vi "Day_File_Plotter.vi"() -> ()   [LabVIEW 2010]
uses:
  Anemometry/Anemometry Sub Vis/Globals/Constants_global.vi
panel:
  in  "Reload":bool
  out "Setup exists?":bool
  out "Plot 3 status":string
  out "Plot 2 status":string
  out "Plot 1 status":string
  out "Change Scale?":bool
  out "Min Memory":timestamp
  out "Max Memory":timestamp
  in  "Show Full Time?":bool
  in  "Max Time":timestamp format="%<%H:%M\n%x>T"
  in  "Min Time":timestamp format="%<%H:%M\n%x>T"
  out "Plot 3 Chs":string[](array[string])
  out "Plot 2 Chs":string[](array[string])
  out "Plot 1 Chs":string[](array[string])
  in  "Save plot number":T1(ring)
  in  "Data folder location":path
  in  "Save 3":bool
  in  "Save 2":bool
  in  "Save 1":bool
  in  "Averaging Time (min)":dbl=1.0 min=0.0 format="%#.2f"
  in  "End Date":timestamp format="%<%x>T"
  in  "Selector 1":i32[](listbox)
  in  "Search 1":string
  in  "Search 2":string
  in  "Search 3":string
  out "Last Updated":string
  out "Plot 3":cluster{"Times":dbl[], "Output array":dbl[]}[](graph)
  in  "Selector 3":i32[](listbox)
  out "Plot 2":cluster{"Times":dbl[], "Output array":dbl[]}[](graph)
  in  "Selector 2":i32[](listbox)
  in  "stop":bool
  out "Plot 1":cluster{dbl[], "Output array":dbl[]}[](graph)
  in  "History (days)":i32 min=0
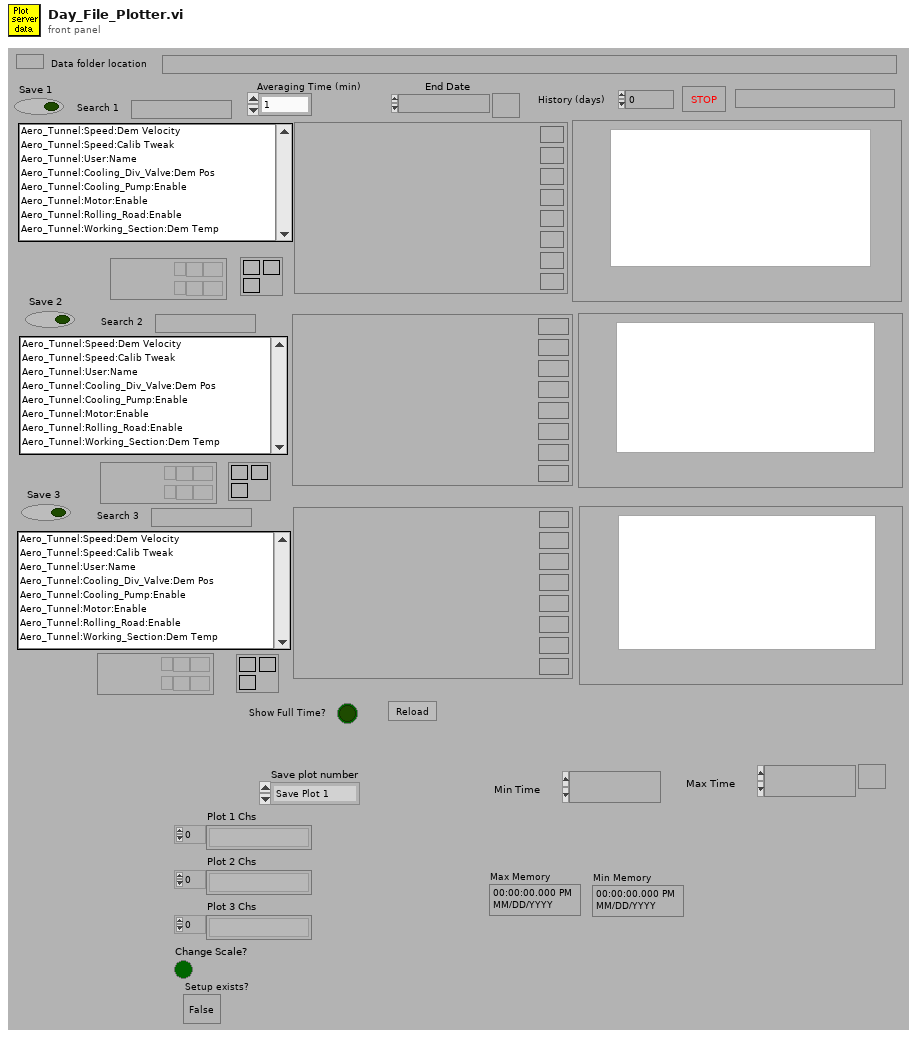
[diagram p1: front panel]
types:
  T1 = enum16{"Save Plot 1", "Save Plot 2", "Save Plot 3"}
  T2 = enum32{"existing file", "new file", "new or existing file", "existing dir", "new dir", "new or existing dir", "existing file (use LLBs)", "new file (use LLBs)", "new or existing file (use LLBs)", "new or existing file or directory (use LLBs)"}
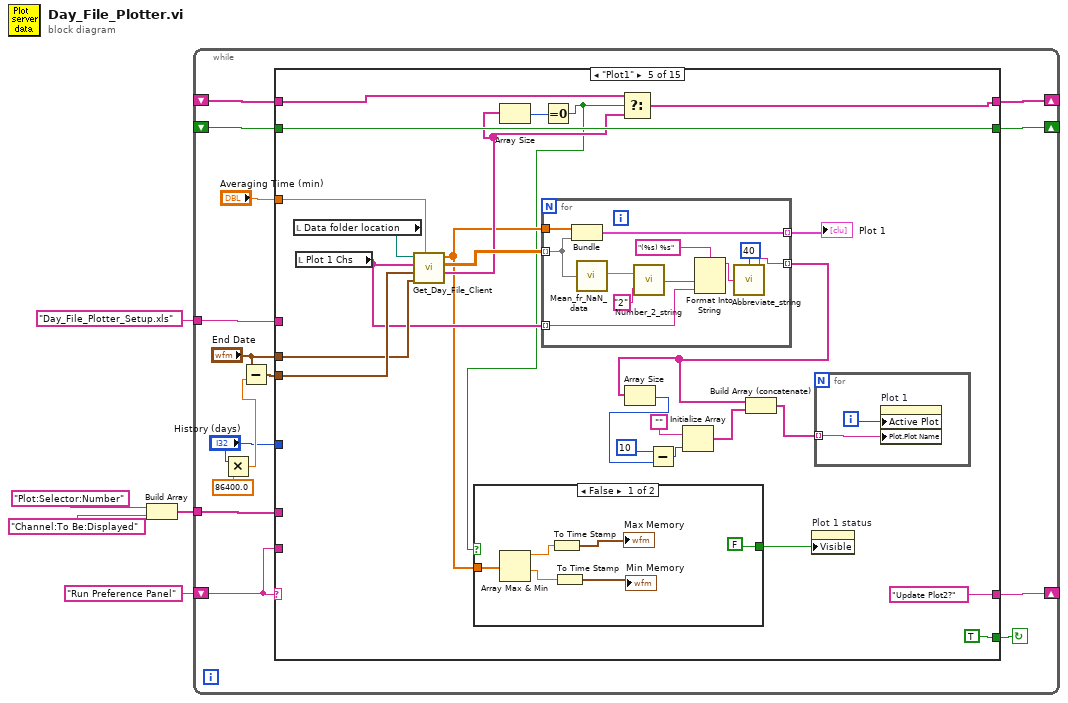
[diagram p0: block diagram]
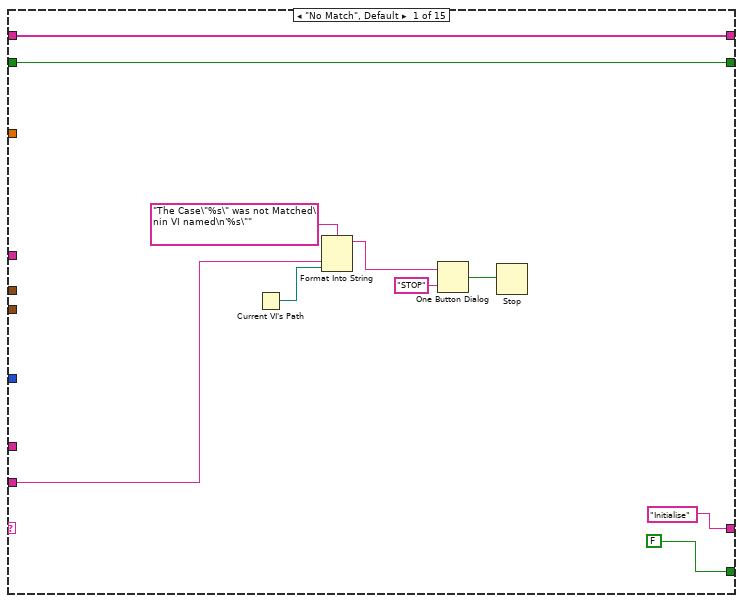
[diagram p2: hidden frame]
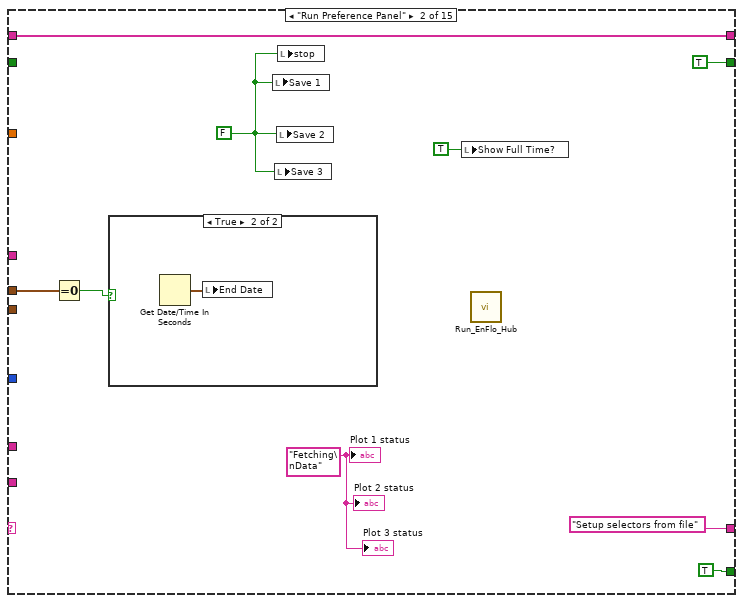
[diagram p3: hidden frame]
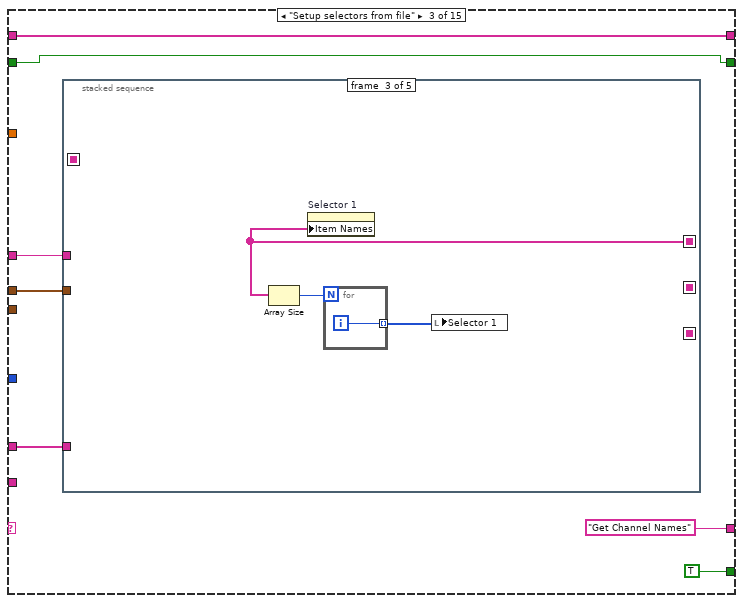
[diagram p5: hidden frame]
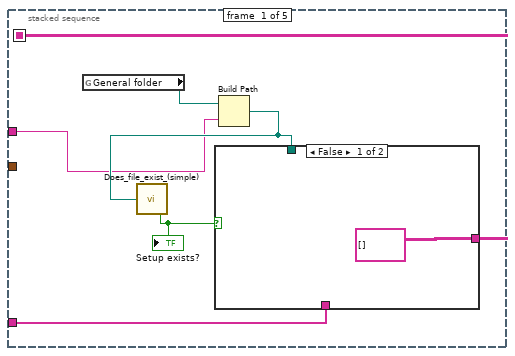
[diagram p6: hidden frame]
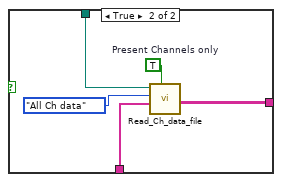
[diagram p7: hidden frame]
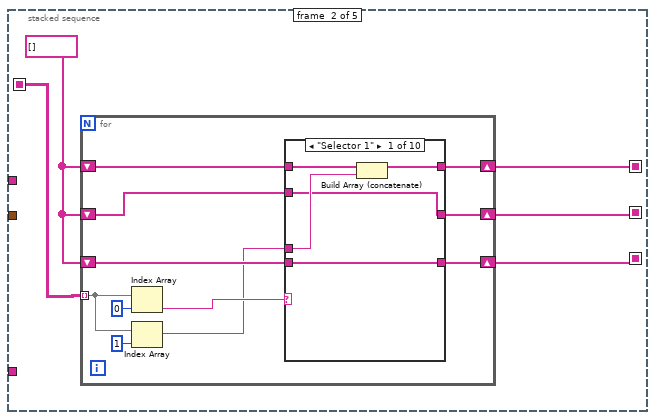
[diagram p8: hidden frame]
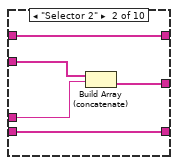
[diagram p9: hidden frame]
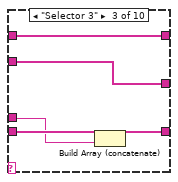
[diagram p10: hidden frame]
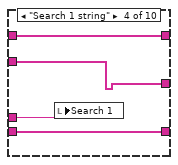
[diagram p11: hidden frame]
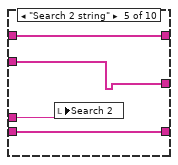
[diagram p12: hidden frame]
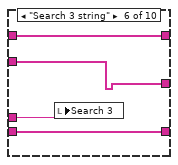
[diagram p13: hidden frame]
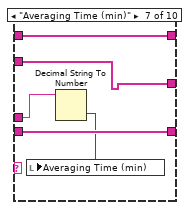
[diagram p14: hidden frame]
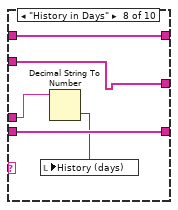
[diagram p15: hidden frame]
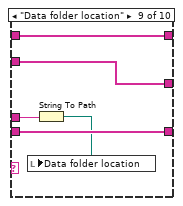
[diagram p16: hidden frame]
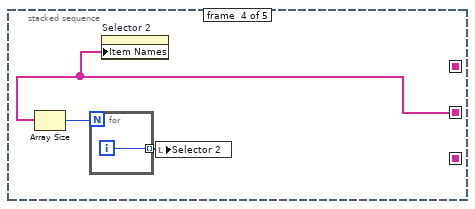
[diagram p18: hidden frame]
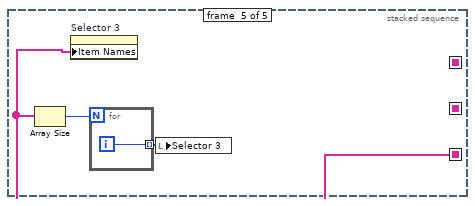
[diagram p19: hidden frame]
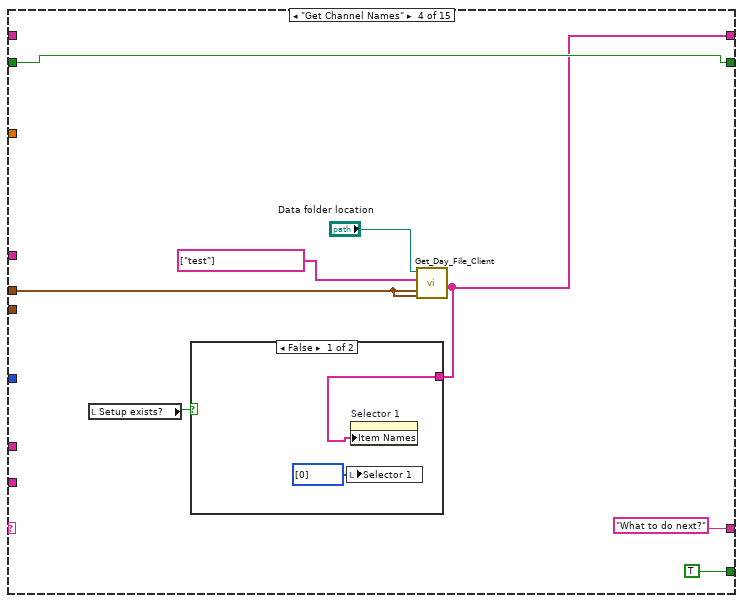
[diagram p20: hidden frame]
diagram:
  n1 = Build Array("Plot:Selector:Number", "Channel:To Be:Displayed") -> (w2:string[])
  n2 = while {
    shift-left: "Run Preference Panel" -> [w18]
    shift-right: [w19] -> _
    tunnel: w2 -> [w17]
    tunnel: "Day_File_Plotter_Setup.xls" -> [w16]
    shift-right: [w11] -> _
    shift-left: _ -> [w10]
    shift-right: [w7] -> _
    shift-left: _ -> [w6]
    stop <- w20 continue-if-true
    n3 = Multiply(x="History (days)", y=86400.0) -> (x*y=w14:dbl)
    n4 = Subtract(x="End Date", y=w14) -> (x-y=w13:timestamp)
    n5 = case shown="\"Plot1\"" w18 {
      tunnel: [FALSE TRUE TRUE TRUE TRUE TRUE TRUE TRUE TRUE TRUE TRUE TRUE TRUE TRUE w605] -> w20
      tunnel: ["Initialise" "Setup selectors from file" "Get Channel Names" "What to do next?" "Update Plot2?" "Update Plot3?" "Rescale plots?" "Update Plot1?" w314 w365 w418 w469 w565 w588 "Check for Zoom" ("t")] -> w19
      tunnel: w18 -> [w25 _ _ _ _ _ _ _ _ _ _ _ _ _ _]
      tunnel: w17 -> [_ _ w44 _ _ _ _ _ _ _ _ _ _ _ w612]
      tunnel: w16 -> [_ _ w45 _ _ _ _ _ _ _ _ _ _ _ w611]
      tunnel: w13 -> [_ _ _ _ w161 w206 w251 _ _ _ _ _ _ _ _]
      tunnel: "End Date" -> [_ w36 w42 w137 w160 w205 w250 _ _ _ _ _ w558 _ _]
      tunnel: [w22 TRUE w43 w138 w164 w209 w254 w282 w331 w383 w435 w470 w557 w587 w609] -> w11
      tunnel: w10 -> [w22 _ w43 w138 w164 w209 w254 w282 w331 w383 w435 w470 _ w586 w609]
      tunnel: "History (days)" -> [_ _ _ _ _ _ _ _ _ _ _ _ _ _ w603]
      tunnel: "Averaging Time (min)" -> [_ _ _ _ w163 w208 w253 _ _ _ _ _ w556 _ w608]
      tunnel: [w21 w34 w41 w134 w155 w200 w245 w283 w327 w379 w431 w471 w554 w593 w607] -> w7
      tunnel: w6 -> [w21 w34 w41 _ w157 w202 w247 w283 w327 w379 w431 w471 w554 w593 w607]
      frame "No Match", Default {
        n6 = Current VI's Path() -> (path=w24:path)
        n7 = Format Into String(format string="The Case\"%s\" was not Matched\nin VI named\n'%s\"" ("Format String"), w25, w24) -> (resulting string=w28:string)  [unwired: 2 in, 1 out]
        n8 = One Button Dialog(message=w28, button name ("OK")="STOP") -> (true=w26:bool)
        n9 = Stop(stop? (T)=w26) -> ()
      }
      frame "Run Preference Panel" {
        w31 = "Fetching\nData" ("Plot 1 status")
        w33 = FALSE
        n10 = Equal To 0?(x=w36) -> (x = 0?=w35:bool)
        n11 = case shown="True" w35 {
          frame False {
          }
          frame True {
            n12 = Get Date/Time In Seconds() -> (seconds since 1Jan1904=w40:timestamp)
            n13 = local write "End Date"(w40) -> ()
          }
        }
        n14 = local write "Save 1"(w33) -> ()
        n15 = local write "Save 3"(w33) -> ()
        n16 = local write "Save 2"(w33) -> ()
        n17 = local write "stop"(w33) -> ()
        n18 = local write "Show Full Time?"(TRUE ("Show Full Time?")) -> ()
        n19 = call "Run_EnFlo_Hub.vi"() -> ()  [unwired: 8 out]
        "Plot 1 status" <- w31
        "Plot 3 status" <- w31
        "Plot 2 status" <- w31
      }
      frame "Setup selectors from file" {
        n20 = stacked-sequence {
          seq-local: [w49 _ _ _ _] -> [_ w64 _ _ _]
          seq-local: [_ w62 _ _ _] -> [_ _ w123 _ _]
          seq-local: [_ w60 _ _ _] -> [_ _ _ w125 _]
          seq-local: [_ w61 _ _ _] -> [_ _ _ _ w129]
          tunnel: w45 -> [w51 _ _ _ _]
          tunnel: w44 -> [w50 _ _ _ _]
          tunnel: w42 -> [_ _ _ _ _]
          frame #0 {
            n21 = global read "Constants_global.vi" "General folder"() -> (w53:path)
            n22 = Build Path(base path=w53, name or relative path=w51) -> (appended path=w52:path)
            n23 = call "Does_file_exist_(simple).vi"("Pathname"=w52) -> ("exists?"=w48:bool)
            "Setup exists?" <- w48
            n24 = case shown="False" w48 {
              tunnel: w52 -> [_ w59]
              tunnel: w50 -> [_ w58]
              tunnel: [string[][] [] ("Channel Values") w55] -> w49
              frame False {
              }
              frame True {
                w57 = TRUE  # Present Channels only
                n25 = call "Read_Ch_data_file.vi"("Present Channels only"=w57, "Present Channels"=w58, "Output"=enum16{"All Ch data", "The last few rows"}."All Ch data", "Filename"=w59) -> ("Channel Values"=w55:string[][])  [unwired: 1 in, 4 out]
              }
            }
          }
          frame #1 {
            w63 = string[] []
            n26 = for {
              shift-right: [w70] -> w62
              shift-left: w63 -> [w71]
              tunnel: w64 -> [w72] mode=indexing
              shift-right: [w68] -> w60
              shift-left: w63 -> [w69]
              shift-right: [w66] -> w61
              shift-left: w63 -> [w67]
              n27 = Index Array(array=w72, index=0 ("Index")) -> (element=w74:string)
              n28 = Index Array(array=w72, index=1 ("Index")) -> (element=w65:string)
              n29 = case shown="\"Selector 1\"" w74 {
                tunnel: w71 -> [w80 w85 w86 w94 w98 w102 w107 w108 w115 w120]
                tunnel: [w79 w85 w86 w94 w98 w102 w107 w108 w115 w120] -> w70
                tunnel: w65 -> [w78 w82 w88 w91 w95 w99 w104 w110 w114 _]
                tunnel: w69 -> [w77 w83 w87 w93 w97 w101 w106 w112 w117 w119]
                tunnel: [w77 w81 w87 w93 w97 w101 w106 w112 w117 w119] -> w68
                tunnel: w67 -> [w76 w84 w90 w92 w96 w100 w105 w111 w116 w118]
                tunnel: [w76 w84 w89 w92 w96 w100 w105 w111 w116 w118] -> w66
                frame "Selector 1" {
                  n30 = Build Array (concatenate)(w80, w78) -> (w79:string[])
                }
                frame "Selector 2" {
                  n31 = Build Array (concatenate)(w83, w82) -> (w81:string[])
                }
                frame "Selector 3" {
                  n32 = Build Array (concatenate)(w90, w88) -> (w89:string[])
                }
                frame "Search 1 string" {
                  n33 = local write "Search 1"(w91) -> ()
                }
                frame "Search 2 string" {
                  n34 = local write "Search 2"(w95) -> ()
                }
                frame "Search 3 string" {
                  n35 = local write "Search 3"(w99) -> ()
                }
                frame "Averaging Time (min)" {
                  n36 = Decimal String To Number(string=w104) -> (number=w103:i32)  [unwired: 3 out]
                  n37 = local write "Averaging Time (min)"(w103) -> ()
                }
                frame "History in Days" {
                  n38 = Decimal String To Number(string=w110) -> (number=w109:i32)  [unwired: 3 out]
                  n39 = local write "History (days)"(w109) -> ()
                }
                frame "Data folder location" {
                  n40 = String To Path(string=w114) -> (path=w113:path)
                  n41 = local write "Data folder location"(w113) -> ()
                }
                frame "No match", Default {
                }
              }
            }
          }
          frame #2 {
            n42 = Array Size(array=w123) -> (size(s)=w122:i32)
            n43 = property on="Selector 1" class="LstBox (strict)"("Item Names"=w123) -> ()  [unwired: 2 in, 2 out]
            n44 = for {
              N: w122 -> [_]
              tunnel: [w124] -> w121 mode=indexing
              i -> [w124]
            }
            n45 = local write "Selector 1"(w121) -> ()
          }
          frame #3 {
            n46 = Array Size(array=w125) -> (size(s)=w127:i32)
            n47 = for {
              N: w127 -> [_]
              tunnel: [w128] -> w126 mode=indexing
              i -> [w128]
            }
            n48 = property on="Selector 2" class="LstBox (strict)"("Item Names"=w125) -> ()  [unwired: 2 in, 2 out]
            n49 = local write "Selector 2"(w126) -> ()
          }
          frame #4 {
            n50 = Array Size(array=w129) -> (size(s)=w131:i32)
            n51 = property on="Selector 3" class="LstBox (strict)"("Item Names"=w129) -> ()  [unwired: 2 in, 2 out]
            n52 = for {
              N: w131 -> [_]
              tunnel: [w132] -> w130 mode=indexing
              i -> [w132]
            }
            n53 = local write "Selector 3"(w130) -> ()
          }
        }
      }
      frame "Get Channel Names" {
        n54 = local read "Setup exists?"() -> (w133:bool)
        n55 = call "Get_Day_File_Client.vi"("End time"=w137, "Start time"=w137, "Channel Names"=string[] ["test"], "Data folder location"="Data folder location") -> ("All Channel Names"=w134:string[])  [unwired: 1 in, 3 out]
        n56 = case shown="False" w133 {
          tunnel: w134 -> [w142 _]
          frame False {
            n57 = local write "Selector 1"(i32[] [0] ("Selector 1")) -> ()
            n58 = property on="Selector 1" class="LstBox (strict)"("Item Names"=w142) -> ()  [unwired: 2 in, 2 out]
          }
          frame True {
          }
        }
      }
      frame "Plot1" {
        n59 = local read "Data folder location"() -> (w162:path)
        n60 = local read "Plot 1 Chs"() -> (w147:string[])
        n61 = call "Get_Day_File_Client.vi"("Averaging Time (min)"=w163, "End time"=w160, "Start time"=w161, "Channel Names"=w147, "Data folder location"=w162) -> ("All Channel Names"=w156:string[], "Data"=w159:dbl[][], "Times"=w145:dbl[])  [unwired: 1 out]
        n62 = Array Size(array=w156) -> (size(s)=w158:i32)
        n63 = for {
          tunnel: w159 -> [w175] mode=indexing
          tunnel: [w184] -> w154 mode=indexing
          tunnel: w145 -> [w183]
          tunnel: [w179] -> w146 mode=indexing
          tunnel: w147 -> [w176] mode=indexing
          n64 = Bundle("Times"=w183, "Data"=w175) -> (w184:cluster{"Times":dbl[], "Data":dbl[]})  [unwired: 1 out]
          n65 = call "Mean_fr_NaN_data.vi"("Data"=w175) -> ("Mean value"=w174:dbl)
          n66 = call "Number_2_string.vi"("precision"="2", "number"=w174) -> ("String"=w177:string)
          n67 = Format Into String(format string="(%s) %s", w177, w176) -> (resulting string=w180:string)  [unwired: 2 in, 1 out]
          n68 = call "Abbreviate_string.vi"("Input String"=w180, "Max String Length"=40) -> ("Output String"=w179:string)
        }
        "Plot 1" <- w154
        n69 = Equal To 0?(x=w158) -> (x = 0?=w144:bool)
        n70 = case shown="False" w144 {
          tunnel: w145 -> [w172 _]
          tunnel: [FALSE ("Visible") FALSE ("Visible")] -> w143
          frame False {
            n71 = Array Max & Min(array=w172) -> (max value=w171:dbl, min value=w169:dbl)  [unwired: 2 out]
            n72 = To Time Stamp(1:w171) -> (0:→"Max Memory":timestamp)
            n73 = To Time Stamp(1:w169) -> (0:→"Min Memory":timestamp)
          }
          frame True {
          }
        }
        n74 = Select(t=w157, s=w144, f=w156) -> (s? t:f=w155:string[])
        n75 = Array Size(array=w146) -> (size(s)=w152:i32)
        n76 = Subtract(x=10 ("dimension size"), y=w152) -> (x-y=w153:i32)
        n77 = Initialize Array("", w153) -> (w150:string[])
        n78 = Build Array (concatenate)(w146, w150) -> (w148:string[])
        n79 = property on="Plot 1 status" class="Str"("Visible"=w143) -> ()  [unwired: 2 in, 2 out]
        n80 = for {
          tunnel: w148 -> [w185] mode=indexing
          i -> [w186]
          n81 = property on="Plot 1" class="XYGraph (strict)"("Active Plot"=w186, "Plot.Plot Name"=w185) -> ()  [unwired: 2 in, 2 out]
        }
      }
      frame "Plot2" {
        n82 = local read "Plot 2 Chs"() -> (w193:string[])
        n83 = local read "Data folder location"() -> (w207:path)
        n84 = call "Get_Day_File_Client.vi"("Averaging Time (min)"=w208, "End time"=w205, "Start time"=w206, "Channel Names"=w193, "Data folder location"=w207) -> ("All Channel Names"=w201:string[], "Data"=w204:dbl[][], "Times"=w190:dbl[])  [unwired: 1 out]
        n85 = Array Size(array=w201) -> (size(s)=w203:i32)
        n86 = for {
          tunnel: w204 -> [w220] mode=indexing
          tunnel: [w229] -> w192 mode=indexing
          tunnel: w190 -> [w228]
          tunnel: [w224] -> w191 mode=indexing
          tunnel: w193 -> [w221] mode=indexing
          n87 = Bundle("Times"=w228, "Data"=w220) -> (w229:cluster{"Times":dbl[], "Data":dbl[]})  [unwired: 1 out]
          n88 = call "Mean_fr_NaN_data.vi"("Data"=w220) -> ("Mean value"=w219:dbl)
          n89 = call "Number_2_string.vi"("precision"="2", "number"=w219) -> ("String"=w222:string)
          n90 = Format Into String(format string="(%s) %s", w222, w221) -> (resulting string=w225:string)  [unwired: 2 in, 1 out]
          n91 = call "Abbreviate_string.vi"("Input String"=w225, "Max String Length"=40) -> ("Output String"=w224:string)
        }
        "Plot 2" <- w192
        n92 = Equal To 0?(x=w203) -> (x = 0?=w189:bool)
        n93 = case shown="True" w189 {
          tunnel: w190 -> [w213 _]
          tunnel: [w212 w218] -> w188
          tunnel: FALSE -> [w212 w218]
          frame False {
            n94 = Array Max & Min(array=w213) -> (max value=w217:dbl, min value=w216:dbl)  [unwired: 2 out]
            n95 = To Time Stamp(1:w217) -> (0:w214:timestamp)
            n96 = To Time Stamp(1:w216) -> (0:w215:timestamp)
            n97 = local write "Max Memory"(w214) -> ()
            n98 = local write "Min Memory"(w215) -> ()
          }
          frame True {
          }
        }
        n99 = Array Size(array=w191) -> (size(s)=w198:i32)
        n100 = Select(t=w202, s=w189, f=w201) -> (s? t:f=w200:string[])
        n101 = Subtract(x=10 ("dimension size"), y=w198) -> (x-y=w199:i32)
        n102 = Initialize Array("", w199) -> (w196:string[])
        n103 = Build Array (concatenate)(w191, w196) -> (w194:string[])
        n104 = property on="Plot 2 status" class="Str"("Visible"=w188) -> ()  [unwired: 2 in, 2 out]
        n105 = for {
          tunnel: w194 -> [w230] mode=indexing
          i -> [w231]
          n106 = property on="Plot 2" class="XYGraph (strict)"("Active Plot"=w231, "Plot.Plot Name"=w230) -> ()  [unwired: 2 in, 2 out]
        }
      }
      frame "Plot3" {
        n107 = local read "Plot 3 Chs"() -> (w238:string[])
        n108 = local read "Data folder location"() -> (w252:path)
        n109 = call "Get_Day_File_Client.vi"("Averaging Time (min)"=w253, "End time"=w250, "Start time"=w251, "Channel Names"=w238, "Data folder location"=w252) -> ("All Channel Names"=w246:string[], "Data"=w249:dbl[][], "Times"=w235:dbl[])  [unwired: 1 out]
        n110 = Array Size(array=w246) -> (size(s)=w248:i32)
        n111 = for {
          tunnel: w249 -> [w265] mode=indexing
          tunnel: [w274] -> w237 mode=indexing
          tunnel: w235 -> [w273]
          tunnel: [w269] -> w236 mode=indexing
          tunnel: w238 -> [w266] mode=indexing
          n112 = Bundle("Times"=w273, "Data"=w265) -> (w274:cluster{"Times":dbl[], "Data":dbl[]})  [unwired: 1 out]
          n113 = call "Mean_fr_NaN_data.vi"("Data"=w265) -> ("Mean value"=w264:dbl)
          n114 = call "Number_2_string.vi"("precision"="2", "number"=w264) -> ("String"=w267:string)
          n115 = Format Into String(format string="(%s) %s", w267, w266) -> (resulting string=w270:string)  [unwired: 2 in, 1 out]
          n116 = call "Abbreviate_string.vi"("Input String"=w270, "Max String Length"=40) -> ("Output String"=w269:string)
        }
        "Plot 3" <- w237
        n117 = Equal To 0?(x=w248) -> (x = 0?=w234:bool)
        n118 = case shown="True" w234 {
          tunnel: w235 -> [w258 _]
          tunnel: [w257 w263] -> w233
          tunnel: FALSE -> [w257 w263]
          frame False {
            n119 = Array Max & Min(array=w258) -> (max value=w262:dbl, min value=w261:dbl)  [unwired: 2 out]
            n120 = To Time Stamp(1:w262) -> (0:w259:timestamp)
            n121 = To Time Stamp(1:w261) -> (0:w260:timestamp)
            n122 = local write "Max Memory"(w259) -> ()
            n123 = local write "Min Memory"(w260) -> ()
          }
          frame True {
          }
        }
        n124 = Array Size(array=w236) -> (size(s)=w243:i32)
        n125 = Select(t=w247, s=w234, f=w246) -> (s? t:f=w245:string[])
        n126 = Subtract(x=10 ("dimension size"), y=w243) -> (x-y=w244:i32)
        n127 = Initialize Array("", w244) -> (w241:string[])
        n128 = Build Array (concatenate)(w236, w241) -> (w239:string[])
        n129 = property on="Plot 3 status" class="Str"("Visible"=w233) -> ()  [unwired: 2 in, 2 out]
        n130 = for {
          tunnel: w239 -> [w275] mode=indexing
          i -> [w276]
          n131 = property on="Plot 3" class="XYGraph (strict)"("Active Plot"=w276, "Plot.Plot Name"=w275) -> ()  [unwired: 2 in, 2 out]
        }
      }
      frame "Check for Zoom" {
        n132 = local read "Change Scale?"() -> (w278:bool)
        n133 = Or(x=w278, y="Show Full Time?") -> (x .or. y?=w277:bool)
        n134 = case shown="False" w277 {
          frame False {
            n135 = local read "Max Time"() -> (w290:timestamp)
            n136 = local read "Min Time"() -> (w291:timestamp)
            n137 = To Double Precision Float(number=w290) -> (double precision float=w289:dbl)
            n138 = To Double Precision Float(number=w291) -> (double precision float=w288:dbl)
            n139 = while {
              tunnel: w289 -> [w300]
              tunnel: w288 -> [w299]
              tunnel: [w293] -> w287
              tunnel: [w292] -> w286
              i -> [w302]
              stop <- w294 continue-if-true
              n140 = Increment(x=w302) -> (x+1=w301:i32)
              n141 = case shown="3" w301 {
                tunnel: [w305 w307 w310] -> w293
                tunnel: [w304 w306 w309] -> w292
                tunnel: [TRUE TRUE FALSE] -> w295
                frame 1, Default {
                  n142 = property on="Plot 1" class="XYGraph (strict)"() -> ("X Scale.Range:Maximum"=w305:dbl, "X Scale.Range:Minimum"=w304:dbl)  [unwired: 2 in, 2 out]
                }
                frame 2 {
                  n143 = property on="Plot 2" class="XYGraph (strict)"() -> ("X Scale.Range:Maximum"=w307:dbl, "X Scale.Range:Minimum"=w306:dbl)  [unwired: 2 in, 2 out]
                }
                frame 3 {
                  n144 = property on="Plot 3" class="XYGraph (strict)"() -> ("X Scale.Range:Maximum"=w310:dbl, "X Scale.Range:Minimum"=w309:dbl)  [unwired: 2 in, 2 out]
                }
              }
              n145 = Equal?(x=w300, y=w293) -> (x = y?=w297:bool)
              n146 = Equal?(x=w292, y=w299) -> (x = y?=w298:bool)
              n147 = And(x=w297, y=w298) -> (x .and. y?=w296:bool)
              n148 = And(x=w296, y=w295) -> (x .and. y?=w294:bool)
            }
            n149 = To Time Stamp(1:w287) -> (0:w284:timestamp)
            n150 = To Time Stamp(1:w286) -> (0:w285:timestamp)
            n151 = local write "Max Time"(w284) -> ()
            n152 = local write "Min Time"(w285) -> ()
          }
          frame True {
          }
        }
      }
      frame "Update Plot1?" {
        n153 = property on="Selector 1" class="LstBox (strict)"() -> ("Item Names"=w325:string[])  [unwired: 2 in, 2 out]
        n154 = case shown="True" "Save 1" {
          tunnel: ["Update Plot2?" "Save Plot" ("t")] -> w312
          frame False {
          }
          frame True {
            n155 = local write "Save plot number"(T1."Save Plot 1" ("Save plot number")) -> ()
          }
        }
        n156 = for {
          tunnel: w327 -> [w353]
          shift-right: [w348] -> w326
          shift-left: string[] [] -> [w349]
          tunnel: w325 -> [w351]
          tunnel: "Selector 1" -> [w350] mode=indexing
          n157 = Index Array(array=w351, index=w350) -> (element=w347:string)
          n158 = Search 1D Array(1D array=w353, element=w347) -> (index of element=w352:i32)  [unwired: 1 out]
          n159 = case shown="0, Default" w352 {
            tunnel: w352 -> [_ _]
            tunnel: w349 -> [w356 w357]
            tunnel: [w355 w357] -> w348
            tunnel: w347 -> [w354 _]
            frame 0, Default {
              n160 = Build Array (concatenate)(w356, w354) -> (w355:string[])
            }
            frame -1 {
            }
          }
        }
        "Plot 1 Chs" <- w326
        n161 = while {
          shift-right: [w358] -> w334
          shift-left: _ -> [w363]
          tunnel: [w363] -> w333
          shift-right: [w360] -> _
          shift-left: _ -> [w361]
          tunnel: w331 -> [w360]
          tunnel: [w359] -> w330
          tunnel: w326 -> [w358]
          stop <- FALSE continue-if-true
          n162 = Not Equal?(x=w361, y=w360) -> (x != y?=w359:bool)
        }
        n163 = Not Equal?(x=w333, y=w334) -> (x != y?=w332:bool)
        n164 = And(x=w331, y=w330) -> (x .and. y?=w329:bool)
        n165 = Compound Arithmetic op=OR(w329, w332) -> (w313:bool)
        n166 = case shown="True" w313 {
          tunnel: [w336 "Plot1"] -> w314
          tunnel: w312 -> [w336 _]
          frame False {
          }
          frame True {
            n167 = property on="Plot 1 status" class="Str"("Visible"=TRUE) -> ()  [unwired: 2 in, 2 out]
          }
        }
        n168 = call "Selection_with_Search.vi"("Selected Channel Names"=w326, "Search String"="Search 1", "All Channel Names"=w327) -> ("Item Names"=w322:string[])
        n169 = for {
          tunnel: w322 -> [w346]
          tunnel: w326 -> [w345] mode=indexing
          tunnel: [w344] -> w323 mode=indexing
          n170 = Search 1D Array(1D array=w346, element=w345) -> (index of element=w344:i32)  [unwired: 1 out]
        }
        n171 = Not Equal?(x=w322, y=w325) -> (x != y?=w324:bool)
        n172 = To Double Precision Float(number="Max Time") -> (double precision float=w317:dbl)
        n173 = To Double Precision Float(number="Min Time") -> (double precision float=w315:dbl)
        n174 = case shown="True" w324 {
          tunnel: w323 -> [_ w343]
          tunnel: w322 -> [_ w342]
          frame False {
          }
          frame True {
            n175 = local write "Selector 1"(w343) -> ()
            n176 = property on="Selector 1" class="LstBox (strict)"("Item Names"=w342) -> ()  [unwired: 2 in, 2 out]
          }
        }
        n177 = property on="Plot 1" class="XYGraph (strict)"("X Scale.Range:Maximum"=w317, "X Scale.Range:Minimum"=w315) -> ()  [unwired: 2 in, 2 out]
      }
      frame "Update Plot2?" {
        n178 = property on="Selector 2" class="LstBox (strict)"() -> ("Item Names"=w374:string[])  [unwired: 2 in, 2 out]
        n179 = case shown="True" "Save 2" {
          tunnel: ["Update Plot3?" "Save Plot" ("t")] -> w364
          frame False {
          }
          frame True {
            n180 = local write "Save plot number"(T1."Save Plot 2" ("Save plot number")) -> ()
          }
        }
        n181 = for {
          tunnel: w379 -> [w405]
          shift-right: [w400] -> w378
          shift-left: string[] [] -> [w401]
          tunnel: w374 -> [w403]
          tunnel: "Selector 2" -> [w402] mode=indexing
          n182 = Index Array(array=w403, index=w402) -> (element=w399:string)
          n183 = Search 1D Array(1D array=w405, element=w399) -> (index of element=w404:i32)  [unwired: 1 out]
          n184 = case shown="0, Default" w404 {
            tunnel: w404 -> [_ _]
            tunnel: w401 -> [w408 w409]
            tunnel: [w407 w409] -> w400
            tunnel: w399 -> [w406 _]
            frame 0, Default {
              n185 = Build Array (concatenate)(w408, w406) -> (w407:string[])
            }
            frame -1 {
            }
          }
        }
        "Plot 2 Chs" <- w378
        n186 = while {
          shift-right: [w410] -> w386
          shift-left: _ -> [w415]
          tunnel: [w415] -> w385
          shift-right: [w412] -> _
          shift-left: _ -> [w413]
          tunnel: w383 -> [w412]
          tunnel: [w411] -> w382
          tunnel: w378 -> [w410]
          stop <- FALSE continue-if-true
          n187 = Not Equal?(x=w413, y=w412) -> (x != y?=w411:bool)
        }
        n188 = Not Equal?(x=w385, y=w386) -> (x != y?=w384:bool)
        n189 = And(x=w383, y=w382) -> (x .and. y?=w381:bool)
        n190 = local read "Max Time"() -> (w369:timestamp)
        n191 = local read "Min Time"() -> (w370:timestamp)
        n192 = Compound Arithmetic op=OR(w381, w384) -> (w366:bool)
        n193 = To Double Precision Float(number=w369) -> (double precision float=w368:dbl)
        n194 = To Double Precision Float(number=w370) -> (double precision float=w367:dbl)
        n195 = case shown="True" w366 {
          tunnel: [w388 "Plot2"] -> w365
          tunnel: w364 -> [w388 _]
          frame False {
          }
          frame True {
            n196 = property on="Plot 2 status" class="Str"("Visible"=TRUE) -> ()  [unwired: 2 in, 2 out]
          }
        }
        n197 = call "Selection_with_Search.vi"("Selected Channel Names"=w378, "Search String"="Search 2", "All Channel Names"=w379) -> ("Item Names"=w375:string[])
        n198 = for {
          tunnel: w375 -> [w398]
          tunnel: w378 -> [w397] mode=indexing
          tunnel: [w396] -> w376 mode=indexing
          n199 = Search 1D Array(1D array=w398, element=w397) -> (index of element=w396:i32)  [unwired: 1 out]
        }
        n200 = property on="Plot 2" class="XYGraph (strict)"("X Scale.Range:Maximum"=w368, "X Scale.Range:Minimum"=w367) -> ()  [unwired: 2 in, 2 out]
        n201 = Not Equal?(x=w375, y=w374) -> (x != y?=w377:bool)
        n202 = case shown="True" w377 {
          tunnel: w376 -> [_ w395]
          tunnel: w375 -> [_ w394]
          frame False {
          }
          frame True {
            n203 = local write "Selector 2"(w395) -> ()
            n204 = property on="Selector 2" class="LstBox (strict)"("Item Names"=w394) -> ()  [unwired: 2 in, 2 out]
          }
        }
      }
      frame "Update Plot3?" {
        n205 = property on="Selector 3" class="LstBox (strict)"() -> ("Item Names"=w423:string[])  [unwired: 2 in, 2 out]
        n206 = case shown="False" "Save 3" {
          tunnel: ["Rescale plots?" "Save Plot" ("t")] -> w416
          frame False {
          }
          frame True {
            n207 = local write "Save plot number"(T1."Save Plot 3" ("Save plot number")) -> ()
          }
        }
        n208 = for {
          tunnel: w431 -> [w457]
          shift-right: [w452] -> w430
          shift-left: string[] [] -> [w453]
          tunnel: w423 -> [w455]
          tunnel: "Selector 3" -> [w454] mode=indexing
          n209 = Index Array(array=w455, index=w454) -> (element=w451:string)
          n210 = Search 1D Array(1D array=w457, element=w451) -> (index of element=w456:i32)  [unwired: 1 out]
          n211 = case shown="0, Default" w456 {
            tunnel: w456 -> [_ _]
            tunnel: w453 -> [w460 w461]
            tunnel: [w459 w461] -> w452
            tunnel: w451 -> [w458 _]
            frame 0, Default {
              n212 = Build Array (concatenate)(w460, w458) -> (w459:string[])
            }
            frame -1 {
            }
          }
        }
        "Plot 3 Chs" <- w430
        n213 = while {
          shift-right: [w462] -> w438
          shift-left: _ -> [w467]
          tunnel: [w467] -> w437
          shift-right: [w464] -> _
          shift-left: _ -> [w465]
          tunnel: w435 -> [w464]
          tunnel: [w463] -> w434
          tunnel: w430 -> [w462]
          stop <- FALSE continue-if-true
          n214 = Not Equal?(x=w465, y=w464) -> (x != y?=w463:bool)
        }
        n215 = Not Equal?(x=w437, y=w438) -> (x != y?=w436:bool)
        n216 = And(x=w435, y=w434) -> (x .and. y?=w433:bool)
        n217 = Compound Arithmetic op=OR(w433, w436) -> (w417:bool)
        n218 = case shown="True" w417 {
          tunnel: [w440 "Plot3"] -> w418
          tunnel: w416 -> [w440 _]
          frame False {
          }
          frame True {
            n219 = property on="Plot 3 status" class="Str"("Visible"=TRUE) -> ()  [unwired: 2 in, 2 out]
          }
        }
        n220 = local read "Max Time"() -> (w421:timestamp)
        n221 = local read "Min Time"() -> (w422:timestamp)
        n222 = call "Selection_with_Search.vi"("Selected Channel Names"=w430, "Search String"="Search 3", "All Channel Names"=w431) -> ("Item Names"=w427:string[])
        n223 = for {
          tunnel: w427 -> [w450]
          tunnel: w430 -> [w449] mode=indexing
          tunnel: [w448] -> w428 mode=indexing
          n224 = Search 1D Array(1D array=w450, element=w449) -> (index of element=w448:i32)  [unwired: 1 out]
        }
        n225 = Not Equal?(x=w427, y=w423) -> (x != y?=w429:bool)
        n226 = To Double Precision Float(number=w421) -> (double precision float=w420:dbl)
        n227 = To Double Precision Float(number=w422) -> (double precision float=w419:dbl)
        n228 = case shown="True" w429 {
          tunnel: w428 -> [_ w447]
          tunnel: w427 -> [_ w446]
          frame False {
          }
          frame True {
            n229 = local write "Selector 3"(w447) -> ()
            n230 = property on="Selector 3" class="LstBox (strict)"("Item Names"=w446) -> ()  [unwired: 2 in, 2 out]
          }
        }
        n231 = property on="Plot 3" class="XYGraph (strict)"("X Scale.Range:Maximum"=w420, "X Scale.Range:Minimum"=w419) -> ()  [unwired: 2 in, 2 out]
      }
      frame "Save Plot" {
        n232 = stacked-sequence {
          seq-local: [w486 _] -> [_ w522]
          seq-local: [w474 _] -> [_ w524]
          seq-local: [w472 _] -> [_ w523]
          tunnel: ["What to do next?" _] -> w469
          frame #0 {
            n233 = case shown="\"Save Plot 3\"" "Save plot number" {
              tunnel: [w499 w502 w505] -> w491
              tunnel: [w498 w501 w504] -> w486
              frame "Save Plot 1" {
                n234 = local read "Plot 1 Chs"() -> (w498:string[])
                n235 = local write "Save 1"(FALSE ("Save 1")) -> ()
                n236 = local read "Plot 1"() -> (w499:cluster{dbl[], "Output array":dbl[]}[])
              }
              frame "Save Plot 2" {
                n237 = local read "Plot 2 Chs"() -> (w501:string[])
                n238 = local write "Save 2"(FALSE ("Save 1")) -> ()
                n239 = local read "Plot 2"() -> (w502:cluster{"Times":dbl[], "Output array":dbl[]}[])
              }
              frame "Save Plot 3" {
                n240 = local read "Plot 3 Chs"() -> (w504:string[])
                n241 = local write "Save 3"(FALSE ("Save 1")) -> ()
                n242 = local read "Plot 3"() -> (w505:cluster{"Times":dbl[], "Output array":dbl[]}[])
              }
            }
            n243 = local read "Min Time"() -> (w485:timestamp)
            n244 = local read "Max Time"() -> (w483:timestamp)
            n245 = Index Array(array=w491, index=0) -> (element=w489:cluster{"Times":dbl[], "Output array":dbl[]})
            n246 = To Double Precision Float(number=w485) -> (double precision float=w481:dbl)
            n247 = To Double Precision Float(number=w483) -> (double precision float=w482:dbl)
            n248 = Unbundle(w489) -> ("Times"=w475:dbl[])  [unwired: 1 out]
            n249 = Threshold 1D Array(2:w481, 3:w475) -> (0:w484:dbl)  [unwired: 1 out]
            n250 = Threshold 1D Array(2:w482, 3:w475) -> (0:w480:dbl)  [unwired: 1 out]
            n251 = Round Toward -Infinity(1:w484) -> (0:w478:dbl)
            n252 = Round Toward +Infinity(x=w480) -> (ceil(x): smallest int >= x=w479:dbl)
            n253 = To Long Integer(number=w478) -> (32bit integer=w477:i32)
            n254 = Subtract(x=w479, y=w478) -> (x-y=w476:dbl)
            n255 = for {
              N: w476 -> [_]
              tunnel: w477 -> [w496]
              tunnel: w475 -> [w494]
              tunnel: [w493] -> w474 mode=indexing
              tunnel: [w492] -> w473 mode=indexing
              i -> [w495]
              n256 = Add(x=w496, y=w495) -> (x+y=w492:i32)
              n257 = Index Array(array=w494, index=w492) -> (element=w493:dbl)
            }
            n258 = for {
              tunnel: w491 -> [w509] mode=indexing
              tunnel: w473 -> [w508]
              tunnel: [w506] -> w472 mode=indexing
              n259 = Unbundle(w509) -> ("Output array"=w507:dbl[])  [unwired: 1 out]
              n260 = for {
                tunnel: w508 -> [w512] mode=indexing
                tunnel: w507 -> [w511]
                tunnel: [w510] -> w506 mode=indexing
                n261 = Index Array(array=w511, index=w512) -> (element=w510:dbl)
              }
            }
          }
          frame #1 {
            w517 = FALSE  # append to file? (new file:F)
            (unwired) T2."new file" ("select mode (2)")
            n262 = for {
              tunnel: w523 -> [w541]
              tunnel: w524 -> [w535] mode=indexing
              tunnel: [w537] -> w516 mode=indexing
              i -> [w540]
              n263 = Number To Decimal String(number=w535) -> (decimal integer string=w536:string)  [unwired: 1 out]
              n264 = Index Array(array=w541, index (col)=w540) -> (element=w539:dbl[])  [unwired: 1 in]
              n265 = Get Date/Time String(seconds (now)=w535) -> (date string=w534:string, time string=w533:string)  [unwired: 2 out]
              n266 = for {
                tunnel: w539 -> [w543] mode=indexing
                tunnel: [w542] -> w538 mode=indexing
                n267 = call "Number_2_string.vi"("number"=w543) -> ("String"=w542:string)  [unwired: 1 in]
              }
              n268 = Build Array (concatenate)(w534, w533, w536, w538) -> (w537:string[])
            }
            n269 = Build Array (concatenate)("Date::", "Centre:Time:", "Seconds:Since:1st Jan 1904", w522) -> (w515:string[])
            n270 = call "Ch_names_to_rows.vi"("Channel Names"=w515) -> ("3 Row names"=w521:string[][])
            n271 = File Dialog(7:"Please choose file name" ("prompt")) -> (3:w529:path)  [unwired: 1 in, 8 out]
            n272 = Build Array (concatenate)(w521, w516) -> (w519:string[][])
            n273 = Strip Path(path=w529) -> (stripped path=w526:path, name=w528:string)
            n274 = call "Add_filename_suffix.vi"("Filename"=w528, "Suffix to add"=".xls") -> ("Filename out"=w525:string)  [unwired: 3 out]
            n275 = Array To Spreadsheet String(array=w519, 3:"%s" ("format string")) -> (spreadsheet string=w518:string)  [unwired: 1 out]
            n276 = Build Path(base path=w526, name or relative path=w525) -> (appended path=w514:path)
            n277 = call "Write_File_Simple.vi"("append to file? (new file:F)"=w517, "character string"=w518, "file path"=w514) -> ()  [unwired: 2 out]
          }
        }
      }
      frame "What to do next?" {
        n278 = while {
          shift-right: [w581] -> _
          shift-left: _ -> [w580]
          shift-right: [w577] -> _
          shift-left: _ -> [w578]
          tunnel: w556 -> [w577]
          shift-right: [w575] -> _
          shift-left: _ -> [w576]
          tunnel: w558 -> [w575]
          tunnel: [w573] -> w557
          shift-right: [w571] -> w548
          shift-left: _ -> [w572]
          stop <- FALSE continue-if-true
          n279 = local read "History (days)"() -> (w581:i32)
          n280 = Not Equal?(x=w581, y=w580) -> (x != y?=w570:bool)
          n281 = Not Equal?(x=w577, y=w578) -> (x != y?=w574:bool)
          n282 = Not Equal?(x=w576, y=w575) -> (x != y?=w569:bool)
          n283 = Compound Arithmetic op=OR(w570, w574, w569, "Reload") -> (w573:bool)
          n284 = case shown="False" w573 {
            tunnel: w572 -> [w582 w585]
            tunnel: [w583 w585] -> w571
            frame False {
              n285 = Wait (ms)(milliseconds to wait=u32 100) -> ()  [unwired: 1 out]
              n286 = Increment(x=w582) -> (x+1=w583:dbl)
            }
            frame True {
            }
          }
          n287 = Compound Arithmetic op=OR(w570, w569, "Reload") -> (→"Change Scale?":bool)
        }
        n288 = Get Date/Time String(date format (0)=enum16{"short", "long", "abbreviated"}."abbreviated") -> (date string=w561:string, time string=w562:string)  [unwired: 2 out]
        n289 = Concatenate Strings(w561, " at " ("Substring"), w562) -> (→"Last Updated":string)
        n290 = Array Size(array=w554) -> (size(s)=w555:i32)
        n291 = Greater Than 0?(x=w555) -> (x > 0?=w553:bool)
        n292 = Select(t="Check for Zoom", s=w553, f="Get Channel Names") -> (s? t:f=w550:string)
        n293 = Quotient & Remainder(x=w548, y=500) -> (x-y*floor(x/y)=w547:i32)  [unwired: 1 out]
        n294 = Equal To 0?(x=w547) -> (x = 0?=w545:bool)
        n295 = Or(x=w545, y="stop") -> (x .or. y?=w544:bool)
        n296 = Select(t="Save Channel Names", s=w544, f=w550) -> (s? t:f=w565:string)
      }
      frame "Rescale plots?" {
        n297 = local read "Show Full Time?"() -> (w589:bool)
        n298 = local read "Change Scale?"() -> (w591:bool)
        n299 = Or(x=w591, y=w589) -> (x .or. y?=w590:bool)
        n300 = case shown="False" w590 {
          tunnel: ["What to do next?" "Update Plot1?"] -> w588
          tunnel: [w594 FALSE] -> w587
          tunnel: w586 -> [w594 _]
          frame False {
          }
          frame True {
            w597 = FALSE ("Show Full Time?")
            n301 = local write "Show Full Time?"(w597) -> ()
            n302 = local write "Change Scale?"(w597) -> ()
            n303 = local read "Max Memory"() -> (w599:timestamp)
            n304 = local read "Min Memory"() -> (w600:timestamp)
            n305 = local write "Max Time"(w599) -> ()
            n306 = local write "Min Time"(w600) -> ()
          }
        }
      }
      frame "Save Channel Names" {
        w602 = 10 ("y")
        n307 = Less?(x=w603, y=w602) -> (x < y?=w604:bool)
        n308 = global read "Constants_global.vi" "General folder"() -> (w601:path)
        n309 = stacked-sequence {
          seq-local: [w614 _ _] -> [_ w656 _]
          seq-local: [_ w653 _] -> [_ _ w664]
          tunnel: w612 -> [_ _ w665]
          tunnel: w611 -> [_ _ w668]
          tunnel: w608 -> [_ w652 _]
          tunnel: w604 -> [_ w640 _]
          tunnel: w603 -> [_ w639 _]
          tunnel: w602 -> [_ w638 _]
          tunnel: w601 -> [_ _ w667]
          frame #0 {
            n310 = for {
              N: 3 -> [_]
              shift-right: [w618] -> w614
              shift-left: string[][] [] -> [w620]
              i -> [w625]
              n311 = Increment(x=w625) -> (x+1=w622:i32)
              n312 = case shown="2" w622 {
                tunnel: [w632 w633 w635] -> w624
                tunnel: [w631 w634 w636] -> w616
                frame 1, Default {
                  n313 = local read "Selector 1"() -> (w632:i32[])
                  n314 = property on="Selector 1" class="LstBox (strict)"() -> ("Item Names"=w631:string[])  [unwired: 2 in, 2 out]
                }
                frame 2 {
                  n315 = property on="Selector 2" class="LstBox (strict)"() -> ("Item Names"=w634:string[])  [unwired: 2 in, 2 out]
                  n316 = local read "Selector 2"() -> (w633:i32[])
                }
                frame 3 {
                  n317 = local read "Selector 3"() -> (w635:i32[])
                  n318 = property on="Selector 3" class="LstBox (strict)"() -> ("Item Names"=w636:string[])  [unwired: 2 in, 2 out]
                }
              }
              n319 = Format Into String(format string="%d" ("Format String"), initial string="Selector ", w622) -> (resulting string=w619:string)  [unwired: 1 in, 1 out]
              n320 = for {
                tunnel: w624 -> [w630] mode=indexing
                tunnel: w619 -> [w629]
                tunnel: [w627] -> w617 mode=indexing
                tunnel: w616 -> [w626]
                n321 = Index Array(array=w626, index=w630) -> (element=w628:string)
                n322 = Build Array(w629, w628) -> (w627:string[])
              }
              n323 = Build Array (concatenate)(w620, w617) -> (w618:string[][])
            }
          }
          frame #1 {
            n324 = Select(t=w639, s=w640, f=w638) -> (s? t:f=w637:i32)
            n325 = local read "Data folder location"() -> (w643:path)
            n326 = local read "Search 1"() -> (w662:string)
            n327 = Number To Decimal String(number=w652) -> (decimal integer string=w650:string)  [unwired: 1 out]
            n328 = local read "Search 2"() -> (w659:string)
            n329 = Number To Decimal String(number=w637) -> (decimal integer string=w647:string)  [unwired: 1 out]
            n330 = local read "Search 3"() -> (w658:string)
            n331 = Path To String(path=w643) -> (string=w642:string)
            n332 = Build Array("Averaging Time (min)" ("element"), w650) -> (w648:string[])
            n333 = Build Array("Search 1 string" ("element"), w662) -> (w649:string[])
            n334 = Build Array("History in Days" ("element"), w647) -> (w645:string[])
            n335 = Build Array("Search 2 string" ("element"), w659) -> (w655:string[])
            n336 = Build Array("Search 3 string" ("element"), w658) -> (w654:string[])
            n337 = Build Array("Data folder location", w642) -> (w641:string[])
            n338 = Build Array (concatenate)(w656, w641, w645, w648, w649, w655, w654) -> (w653:string[][])
          }
          frame #2 {
            n339 = Build Path(base path=w667, name or relative path=w668) -> (appended path=w666:path)
            n340 = Array Size(array=w664) -> (size(s)=w670:i32[])
            n341 = Index Array(array=w670, index=1 ("Index")) -> (element=w669:i32)
            n342 = Not Equal To 0?(x=w669) -> (x != 0?=w663:bool)
            n343 = case shown="True" w663 {
              tunnel: w666 -> [w672 w677]
              tunnel: w664 -> [_ w678]
              tunnel: w665 -> [_ w679]
              frame False {
                n344 = Delete(path (use dialog)=w672) -> ()  [unwired: 1 in, 6 out]
              }
              frame True {
                w673 = FALSE  # append to file? (new file:F)
                n345 = call "Ch_names_to_rows.vi"("Channel Names"=w679) -> ("3 Row names"=w680:string[][])
                n346 = Build Array (concatenate)(w680, w678) -> (w675:string[][])
                n347 = Array To Spreadsheet String(array=w675, 3:"%s" ("format string")) -> (spreadsheet string=w674:string)  [unwired: 1 out]
                n348 = call "Write_File_Simple.vi"("append to file? (new file:F)"=w673, "character string"=w674, "file path"=w677) -> ()  [unwired: 2 out]
              }
            }
          }
        }
        n349 = local read "stop"() -> (w606:bool)
        n350 = Not(x=w606) -> (.not. x?=w605:bool)
      }
    }
  }
